vi "UTEX Simple Send.vi"(7 "UT340 Simple Controls":refnum<vi>, 8 "error in":errorcluster, 9 "Read Back Values?":bool, 10 "Changed Values?":cluster{"PE Gain (dB)":bool, "Voltage":bool}, 11 "UT340 Controls":T1={"PE Gain (dB)"=1, "Voltage"=100} {"Voltage" min=1 max=20 step=1; "PE Gain (dB)" min=-6 max=60 step=1}) -> (0 "error out":errorcluster)   [LabVIEW 2022 SP3]
uses:
  Controls/UTEX Controls Simple.ctl
  PulserGlobals.vi
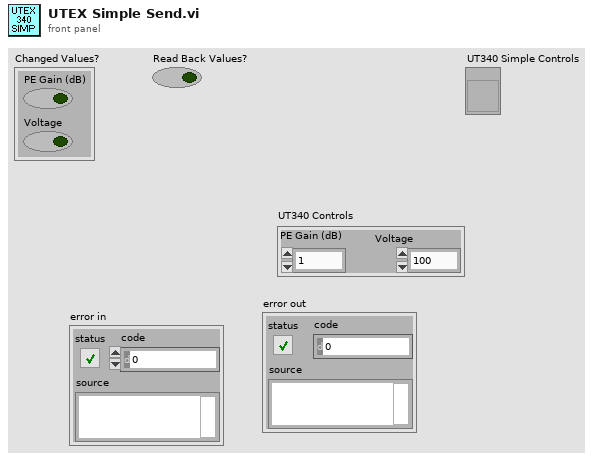
[diagram p1: front panel]
types:
  T1 = typedef "UTEX Controls Simple.ctl" = cluster{"PE Gain (dB)":i16, "Voltage":i16}
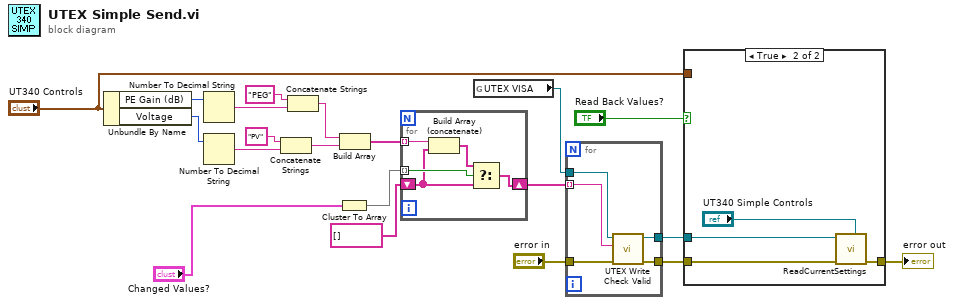
[diagram p0: block diagram]
diagram:
  n1 = Unbundle By Name("UT340 Controls") -> ("PE Gain (dB)"=w18:i16, "Voltage"=w15:i16)
  n2 = Number To Decimal String(number=w18) -> (decimal integer string=w20:string)  [unwired: 1 in]
  n3 = Number To Decimal String(number=w15) -> (decimal integer string=w17:string)  [unwired: 1 in]
  n4 = Concatenate Strings("PV" ("string"), w17) -> (w8:string)
  n5 = Concatenate Strings("PEG" ("string"), w20) -> (w9:string)
  n6 = Cluster To Array(cluster="Changed Values?") -> (array=w13:bool[])
  n7 = Build Array(w9, w8) -> (w10:string[])
  n8 = for {
    tunnel: w13 -> [w25] mode=indexing
    shift-right: [w23] -> w11
    shift-left: string[] [] ("array") -> [w21]
    tunnel: w10 -> [w22] mode=indexing
    n9 = Build Array (concatenate)(w22, w21) -> (w24:string[])
    n10 = Select(t=w24, s=w25, f=w21) -> (s? t:f=w23:string[])
  }
  n11 = global read "PulserGlobals.vi" "UTEX VISA"() -> (w7:refnum<visa-resource-name>)
  n12 = for {
    tunnel: w11 -> [w29] mode=indexing
    tunnel: "error in" -> [w28]
    tunnel: w7 -> [w30]
    tunnel: [w27] -> w4
    tunnel: [w26] -> w6
    n13 = call "UTEX Write Check Valid.vi"("error in"=w28, "write buffer"=w29, "VISA Refnum in"=w30) -> ("error out"=w27:errorcluster, "VISA Refnum out"=w26:refnum<visa-resource-name>)  [unwired: 5 in, 2 out]
  }
  n14 = case shown="True" "Read Back Values?" {
    tunnel: w6 -> [_ w35]
    tunnel: [w31 w34] -> w5
    tunnel: w4 -> [w31 w33]
    tunnel: "UT340 Controls" -> [_ _]
    frame False {
    }
    frame True {
      n15 = call "ReadCurrentSettings.vi"("UT340 Simple Controls"="UT340 Simple Controls", "error in (no error)"=w33, "VISA Refnum in"=w35) -> ("error out"=w34:errorcluster)  [unwired: 6 in, 2 out]
    }
  }
  "error out" <- w5
